vi "Search_Header_Array.vi"(9 "Specific Header":string, 11 "Headers":cluster{"Name":string, "Value":string}[](array[cluster])) -> (3 "Value":string)   [LabVIEW 2016]
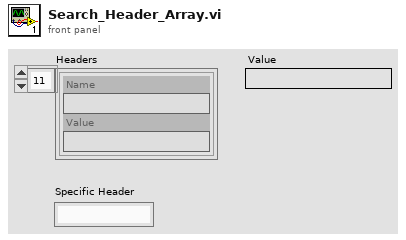
[diagram p1: front panel]
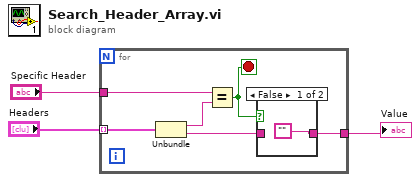
[diagram p0: block diagram]
diagram:
  n1 = for {
    tunnel: "Headers" -> [w9] mode=indexing
    tunnel: "Specific Header" -> [w8]
    tunnel: [w5] -> w1
    stop <- w4 stop-if-true
    n2 = Unbundle(w9) -> ("Name"=w7:string, "Value"=w6:string)
    n3 = Equal?(x=w8, y=w7) -> (x = y?=w4:bool)
    n4 = case shown="False" w4 {
      tunnel: w6 -> [_ w11]
      tunnel: ["" w11] -> w5
      frame False {
      }
      frame True {
      }
    }
  }
  "Value" <- w1
